vi "specu1a 1.0.0 Unit ID to Device Type.vi"(3 "error in":errorcluster, 4 "Unit ID":string) -> (0 "error out":errorcluster, 2 "specu1a 1.0.0 Model Name out":T1)   [LabVIEW 2010]
uses:
  Controls/specu1a 1.0.0 Model Name.ctl
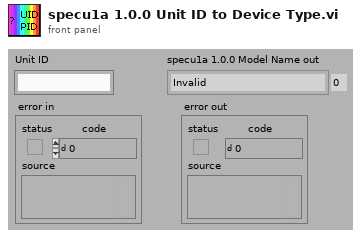
[diagram p1: front panel]
types:
  T1 = typedef "specu1a 1.0.0 Model Name.ctl" = enum16{"Invalid", "TG-NIR", "TG-SWNIR", "TG-UV", "TG-COOLED NIR-II", "TG-COOLED NIR-I", "TM-UV/VIS or VIS/NIR", "TM-UV/VIS or VIS/NIR CCD1", "TM-UV/VIS or VIS/NIR CCD2", "RC-SWNIR Module", "RC-VIS Module"}
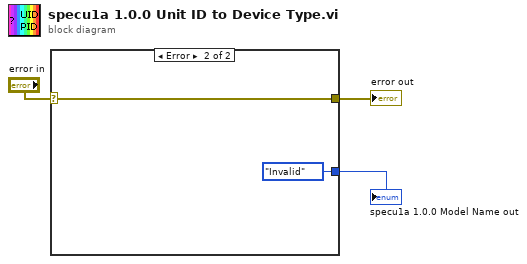
[diagram p0: block diagram]
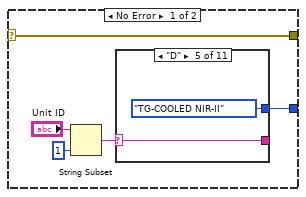
[diagram p2: hidden frame]
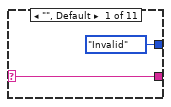
[diagram p3: hidden frame]
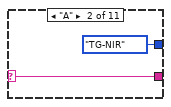
[diagram p4: hidden frame]
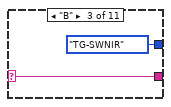
[diagram p5: hidden frame]
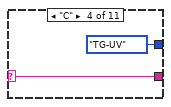
[diagram p6: hidden frame]
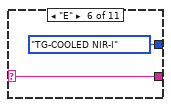
[diagram p7: hidden frame]
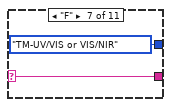
[diagram p8: hidden frame]
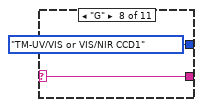
[diagram p9: hidden frame]
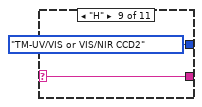
[diagram p10: hidden frame]
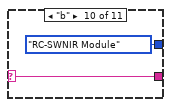
[diagram p11: hidden frame]
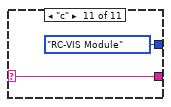
[diagram p12: hidden frame]
diagram:
  n1 = case shown="Error" "error in" {
    selector: "error in" -> [w4 w32]
    tunnel: [w4 w32] -> w3
    tunnel: [w5 specu1a_1.0.0_Model_Name."Invalid" ("specu1a 1.0.0 Model Name out")] -> w1
    frame No Error {
      n2 = String Subset(string="Unit ID", length (rest)=1 ("length (rest)")) -> (substring=w6:string)  [unwired: 1 in]
      n3 = case shown="\"D\"" w6 {
        selector: w6 -> [w9 w12 w14 w16 w18 w20 w22 w24 w26 w28 w30]
        tunnel: [w9 w12 w14 w16 w18 w20 w22 w24 w26 w28 w30] -> _
        tunnel: [specu1a_1.0.0_Model_Name."Invalid" ("specu1a 1.0.0 Model Name out") specu1a_1.0.0_Model_Name."TG-NIR" ("specu1a 1.0.0 Model Name out") specu1a_1.0.0_Model_Name."TG-SWNIR" ("specu1a 1.0.0 Model Name out") specu1a_1.0.0_Model_Name."TG-UV" ("specu1a 1.0.0 Model Name out") specu1a_1.0.0_Model_Name."TG-COOLED NIR-II" ("specu1a 1.0.0 Model Name out") specu1a_1.0.0_Model_Name."TG-COOLED NIR-I" ("specu1a 1.0.0 Model Name out") specu1a_1.0.0_Model_Name."TM-UV/VIS or VIS/NIR" ("specu1a 1.0.0 Model Name out") specu1a_1.0.0_Model_Name."TM-UV/VIS or VIS/NIR CCD1" ("specu1a 1.0.0 Model Name out") specu1a_1.0.0_Model_Name."TM-UV/VIS or VIS/NIR CCD2" ("specu1a 1.0.0 Model Name out") specu1a_1.0.0_Model_Name."RC-SWNIR Module" ("specu1a 1.0.0 Model Name out") specu1a_1.0.0_Model_Name."RC-VIS Module" ("specu1a 1.0.0 Model Name out")] -> w5
        frame "", Default {
        }
        frame "A" {
        }
        frame "B" {
        }
        frame "C" {
        }
        frame "D" {
        }
        frame "E" {
        }
        frame "F" {
        }
        frame "G" {
        }
        frame "H" {
        }
        frame "b" {
        }
        frame "c" {
        }
      }
    }
    frame Error {
    }
  }
  "specu1a 1.0.0 Model Name out" <- w1
  "error out" <- w3
